vi "SPI_Read.vi"(9 "Read Size":u8=1, 10 "Device Register":u8(ring) items=["WHOAMI"=0, "HW_REV"=1, "FW_VER_MAJOR"=2, "FW_VER_MINOR"=3, "UPDATE_RATE_HZ"=4, "ACCEL_FSR_G"=5, "GYRO_FSR_DPS"=6, "OP_STATUS"=8, "CAL_STATUS"=9, "SELFTEST_STATUS"=10, "SENSOR_STATUS"=16, "TIMESTAMP"=18, "YAW"=22, "PITCH"=24, "ROLL"=26, "HEADING"=28, "FUSED_HEADING"=30, "ALTITUDE_I"=32, "ALTITUDE_D"=34, "LINERA_ACC_X"=36, "LINERA_ACC_Y"=38, "LINERA_ACC_Z"=40, "QUAT_W"=42, "QUAT_X"=44, "QUAT_Y"=46, "QUAT_Z"=48, "MPU_TEMP_C"=50, "GYRO_X"=52, "GYRO_Y"=54, "GYRO_Z"=56, "ACC_X"=58, "ACC_Y"=60, "ACC_Z"=62, "MAG_X"=64, "MAG_Y"=66, "MAG_Z"=68, "PRESSURE_I"=70, "PRESSURE_D"=72, "PRESSURE_TEMP"=74, "YAW_OFFSET"=76, "QUAT_OFFSET_W"=78, "QUAT_OFFSET_X"=80, "QUAT_OFFSET_Y"=82, "QUAT_OFFSET_Z"=84], 11 "navX DevRef":T1={"SPIDevRef"={"DevStatus"={"status"=FALSE, "code"=0, "source"=""}, "Handle"=0, "Controller"=enum."Controller 1", "SPI Bus"=enum."SPI On-Board, CS0"}, "Board Information"={"WhoAmI (50 | 0x32)"=0, "Board Revision"=0, "Firmware Major Version"=0, "Firmware Minor Version"=0}, "Status"={"Update Rate Hz"=0, "Accelerometer Full-Scale Range"=0, "Gyro Full-Scale Range"=0, "NAVX_OP_STATUS"=0, "NAVX_CAL_STATUS"=0, "NAVX_SELFTEST_STATUS"=0, "NAVX_SENSOR_STATUS"={"MOVING"=FALSE, "YAW_STABLE"=FALSE, "MAG_DISTURBANCE"=FALSE, "ALTITUDE_VALID"=FALSE, "SEALEVEL_PRESS_SET"=FALSE, "FUSED_HEADING_VALID"=FALSE}}, "Offsets"={"Yaw"=0.0, "Quat W"=0.0, "Quat X"=0.0, "Quat Y"=0.0, "Quat Z"=0.0}, "Update Rate (4Hz-60Hz)"=50, "refnum name"="", "error"={"status"=FALSE, "code"=0, "source"=""}} {"Status"."NAVX_OP_STATUS" items=["INITIALIZING", "SELFTEST_IN_PROGRESS", "ERROR", "IMU_AUTOCAL_IN_PROGRESS", "NORMAL"]; "Status"."NAVX_CAL_STATUS" items=["IMU_CAL_STATE_MASK"=3, "IMU_CAL_INPROGRESS"=0, "IMU_CAL_ACCUMULATE"=1, "IMU_CAL_COMPLETE"=2, "MAG_CAL_COMPLETE"=4, "BARO_CAL_COMPLETE"=8]}) -> (1 "navX Data":u8[](array[numeric]), 2 "Valid?":bool, 3 "navX DevRef":T1={"SPIDevRef"={"DevStatus"={"status"=FALSE, "code"=0, "source"=""}, "Handle"=0, "Controller"=enum."Controller 1", "SPI Bus"=enum."SPI On-Board, CS0"}, "Board Information"={"WhoAmI (50 | 0x32)"=0, "Board Revision"=0, "Firmware Major Version"=0, "Firmware Minor Version"=0}, "Status"={"Update Rate Hz"=0, "Accelerometer Full-Scale Range"=0, "Gyro Full-Scale Range"=0, "NAVX_OP_STATUS"=0, "NAVX_CAL_STATUS"=0, "NAVX_SELFTEST_STATUS"=0, "NAVX_SENSOR_STATUS"={"MOVING"=FALSE, "YAW_STABLE"=FALSE, "MAG_DISTURBANCE"=FALSE, "ALTITUDE_VALID"=FALSE, "SEALEVEL_PRESS_SET"=FALSE, "FUSED_HEADING_VALID"=FALSE}}, "Offsets"={"Yaw"=0.0, "Quat W"=0.0, "Quat X"=0.0, "Quat Y"=0.0, "Quat Z"=0.0}, "Update Rate (4Hz-60Hz)"=50, "refnum name"="", "error"={"status"=FALSE, "code"=0, "source"=""}} {"Status"."NAVX_OP_STATUS" items=["INITIALIZING", "SELFTEST_IN_PROGRESS", "ERROR", "IMU_AUTOCAL_IN_PROGRESS", "NORMAL"]; "Status"."NAVX_CAL_STATUS" items=["IMU_CAL_STATE_MASK"=3, "IMU_CAL_INPROGRESS"=0, "IMU_CAL_ACCUMULATE"=1, "IMU_CAL_COMPLETE"=2, "MAG_CAL_COMPLETE"=4, "BARO_CAL_COMPLETE"=8]})   [LabVIEW 2014, in "navX-MXP IMU.lvlib"]
uses:
  navX-MXP IMU.lvlib
  TypeDefs/navX SPI DevRef.ctl
  <vilib>/Rock Robotics/WPI/SPI/WPI_SPIDevRef.ctl
  <vilib>/Rock Robotics/SystemInterfaces/Typedef/FPGA_TypedefDigitalModule.ctl
  <vilib>/Rock Robotics/SystemInterfaces/spilib/spi_bus.ctl
  COMMON/TypeDefs/navX Board Information.ctl
  COMMON/TypeDefs/navX Status Data.ctl
  COMMON/TypeDefs/navX NAVX_OP_STATUS.ctl
  COMMON/TypeDefs/navX NAVX_CAL_STATUS.ctl
  COMMON/TypeDefs/navX NAVX_SENSOR_STATUS.ctl
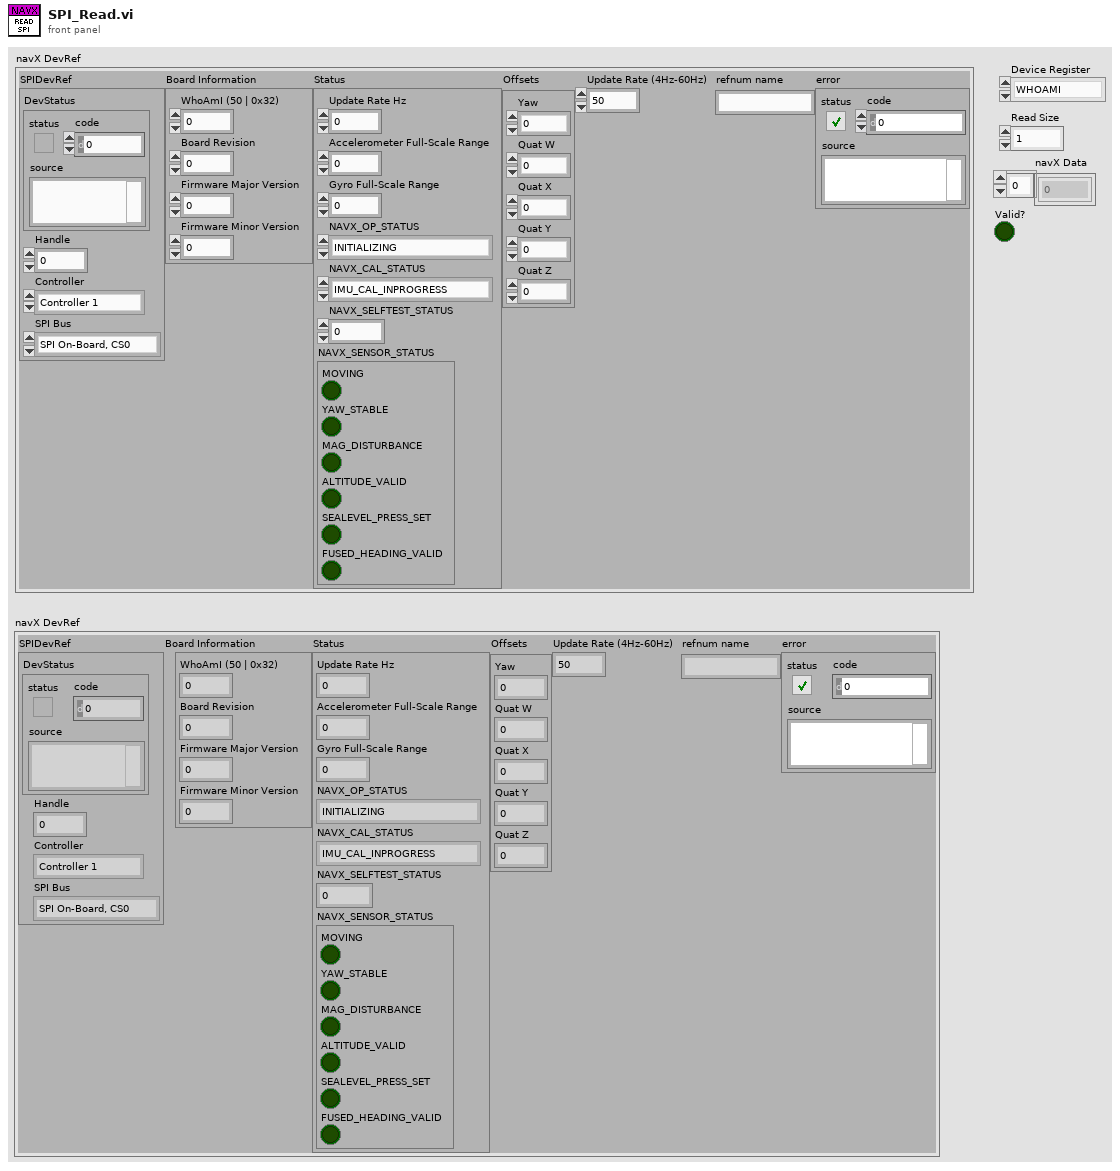
[diagram p1: front panel]
types:
  T1 = typedef "navX-MXP IMU.lvlib/navX SPI DevRef.ctl" = cluster{"SPIDevRef":T2, "Board Information":T5, "Status":T6, "Offsets":cluster{"Yaw":dbl, "Quat W":dbl, "Quat X":dbl, "Quat Y":dbl, "Quat Z":dbl}, "Update Rate (4Hz-60Hz)":u8, "refnum name":string, "error":errorcluster}
  T2 = typedef "WPI_SPIDevRef.ctl" = cluster{"DevStatus":errorcluster, "Handle":i32, "Controller":T3, "SPI Bus":T4}
  T3 = typedef "FPGA_TypedefDigitalModule.ctl" = enum16{"Controller 1"}
  T4 = typedef "spi_bus.ctl" = enum16{"SPI On-Board, CS0", "SPI On-Board, CS1", "SPI On-Board, CS2", "SPI On-Board, CS3", "SPI MXP", "Invalid"}
  T5 = typedef "navX-MXP IMU.lvlib/navX Board Information.ctl" = cluster{"WhoAmI (50 | 0x32)":u8, "Board Revision":u8, "Firmware Major Version":u8, "Firmware Minor Version":u8}
  T6 = typedef "navX-MXP IMU.lvlib/navX Status Data.ctl" = cluster{"Update Rate Hz":u8, "Accelerometer Full-Scale Range":u8, "Gyro Full-Scale Range":u16, "NAVX_OP_STATUS":T7, "NAVX_CAL_STATUS":T8, "NAVX_SELFTEST_STATUS":u8, "NAVX_SENSOR_STATUS":T9}
  T7 = typedef "navX-MXP IMU.lvlib/navX NAVX_OP_STATUS.ctl" = u8
  T8 = typedef "navX-MXP IMU.lvlib/navX NAVX_CAL_STATUS.ctl" = u8
  T9 = typedef "navX-MXP IMU.lvlib/navX NAVX_SENSOR_STATUS.ctl" = cluster{"MOVING":bool, "YAW_STABLE":bool, "MAG_DISTURBANCE":bool, "ALTITUDE_VALID":bool, "SEALEVEL_PRESS_SET":bool, "FUSED_HEADING_VALID":bool}
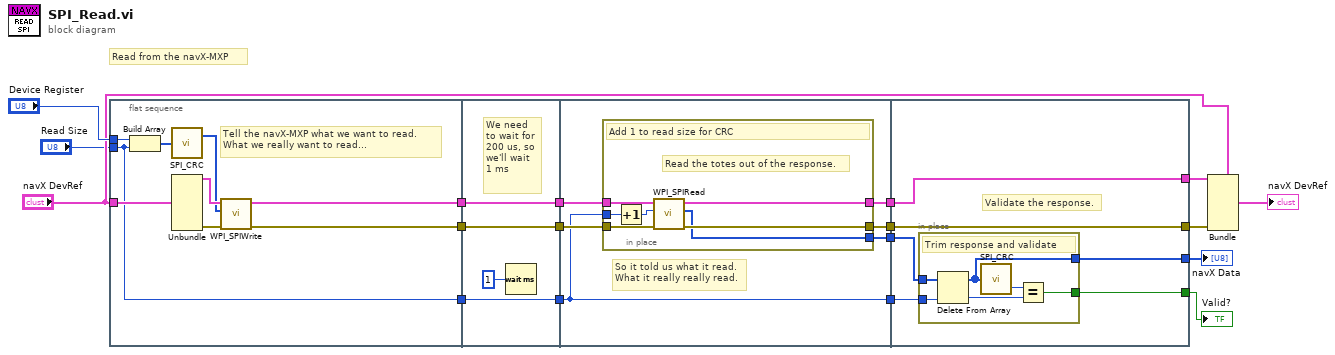
[diagram p0: block diagram]
diagram:
  # "Read from the navX-MXP"
  n1 = flat-sequence {
    tunnel: "Device Register" -> [w23]
    tunnel: "Read Size" -> [w19]
    tunnel: "navX DevRef" -> [w22]
    tunnel: [w21] -> w12
    tunnel: [w20] -> w10
    tunnel: [w19] -> w2
    tunnel: [w30] -> w13
    tunnel: w12 -> [w30]
    tunnel: [w29] -> w11
    tunnel: w10 -> [w29]
    tunnel: [w28] -> w3
    tunnel: w2 -> [w28]
    tunnel: w13 -> [w34]
    tunnel: w11 -> [w33]
    tunnel: [w37] -> w9
    tunnel: [w36] -> w8
    tunnel: [w35] -> w7
    tunnel: w3 -> [w32]
    tunnel: [w32] -> w1
    tunnel: [w49] -> w16
    tunnel: [w50] -> w17
    tunnel: w9 -> [w50]
    tunnel: w8 -> [w48]
    tunnel: w7 -> [w49]
    tunnel: [w47] -> w6
    tunnel: [w46] -> w5
    tunnel: w1 -> [w45]
    frame #0 {
      # "Tell the navX-MXP what we want to read.\nWhat we really want to read..."
      n2 = Build Array(w23, w19) -> (w26:u8[])
      n3 = call "SPI_CRC.vi"("Message"=w26) -> ("Message with CRC"=w24:u8[])  [unwired: 1 out]
      n4 = Unbundle(w22) -> ("SPIDevRef"=w25:T2, "error"=w27:errorcluster)  [unwired: 5 out]
      n5 = call <vilib>:"WPI_SPIWrite.vi"("error in (no error)"=w27, "Data To Send"=w24, "SPIDevRef"=w25) -> ("error out"=w20:errorcluster, "SPIDevRef"=w21:T2)  [unwired: 6 in, 1 out]
    }
    frame #1 {
      # "We need\nto wait for\n200 us, so\nwe'll wait\n1 ms"
      n6 = Wait (ms)(milliseconds to wait=u32 1) -> ()  [unwired: 1 out]
    }
    frame #2 {
      # "So it told us what it read.\nWhat it really really read."
      n7 = in-place {
        in-place-border: w33 -> [w44]
        in-place-border: w34 -> [w43]
        in-place-border: [w42] -> w37
        in-place-border: [w41] -> w35
        in-place-border: [w39] -> w36
        in-place-border: w32 -> [w38]
        # "Read the totes out of the response."
        # "Add 1 to read size for CRC"
        n8 = Increment(x=w38) -> (x+1=w40:u8)
        n9 = call <vilib>:"WPI_SPIRead.vi"("error in (no error)"=w44, "Num to Read"=w40, "SPIDevRef"=w43) -> ("error out"=w41:errorcluster, "Received Data"=w39:u8[], "SPIDevRef"=w42:T2)  [unwired: 6 in]
      }
    }
    frame #3 {
      # "Validate the response."
      n10 = in-place {
        in-place-border: [w55] -> w46
        in-place-border: w48 -> [w54]
        in-place-border: w45 -> [w53]
        in-place-border: [w51] -> w47
        # "Trim response and validate"
        n11 = Delete From Array(array=w54, index=w53) -> (deleted portion=w52:u8, array with subset deleted=w51:u8[])  [unwired: 1 in]
        n12 = call "SPI_CRC.vi"("Message"=w51) -> ("CRC"=w56:u8)  [unwired: 1 out]
        n13 = Equal?(x=w56, y=w52) -> (x = y?=w55:bool)
      }
    }
  }
  n14 = Bundle(cluster="navX DevRef", "SPIDevRef"=w17, "error"=w16) -> (→"navX DevRef":T1)  [unwired: 5 in]
  "navX Data" <- w6
  "Valid?" <- w5
